vi "Create Queue.vi"(8 "error in (no error)":errorcluster) -> (0 "error out":errorcluster, 3 "queue out":refnum<queue>)   [LabVIEW 2014, in "Queues Lib.lvlib"]
uses:
  Queues Lib.lvlib
  Queues Message Type Def.ctl
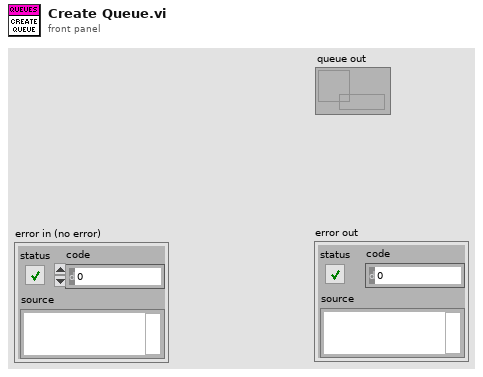
[diagram p1: front panel]
types:
  T1 = typedef "Queues Lib.lvlib/Queues Message Type Def.ctl" = cluster{"Message":string, "Data":variant}
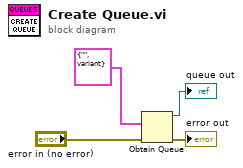
[diagram p0: block diagram]
diagram:
  n1 = Obtain Queue(element data type=T1 {"Message"="", "Data"=variant} ("Queue Message"), error in (no error)="error in (no error)") -> (queue out=→"queue out":refnum<queue>, error out=→"error out":errorcluster)  [unwired: 3 in, 1 out]
